vi "3_june.vi"() -> ()   [LabVIEW 2018]
uses:
  <vilib>/express/express analysis/Spectral/Block/exnSpectralBlock spectral measurements peak poly.vi
  <vilib>/express/express analysis/Spectral/Block/exnSpectralBlock spectral measurements peak DDT.vi
  <vilib>/express/express analysis/Spectral/XNode/ExpressSpectralMeasurementsBlockNode.xnode
panel:
  in  "stop (F)":bool
  out "Orignal Signal":dynamicdata(graph)
  in  "Threshold":dbl=0.1
  out "Portion":dynamicdata(graph)
  in  "Portion Duration":i32=200
  out "Index 0":dbl
  out "Index 1":dbl
  out "Index 2":dbl
  out "Index 3":dbl
  out "dt1":dbl
  out "dt2":dbl
  out "dt3":dbl
  in  "Manual depth":dbl=4.3
  in  "Mode":T1(ring)=enum."Use Far Field"
  out "x":dbl format="%#_6f"
  out "y":dbl format="%#_6f"
  out "z":dbl
  in  "peak min":dbl=0.1
  out "ratio":dbl
  out "ratio 2":dbl
  out "ratio 3":dbl
  out "ratio 4":dbl
  out "amplitude":dbl
  out "amplitude 2":dbl
  out "amplitude 3":dbl
  out "amplitude 4":dbl
  out "yaw":dbl
  out "pitch":dbl
  out "Yaw Chart":dbl(graph)
  out "Freq Domain":dynamicdata(graph)
  out "Ratio at Index (%)":dbl
  in  "LPF Cut-Off":dbl=40000.0 caption="Lower Cut-Off"
  out "Selected Index":i32
  in  "Operating Mode 2":T2(ring)=enum."Analyze Real-time"
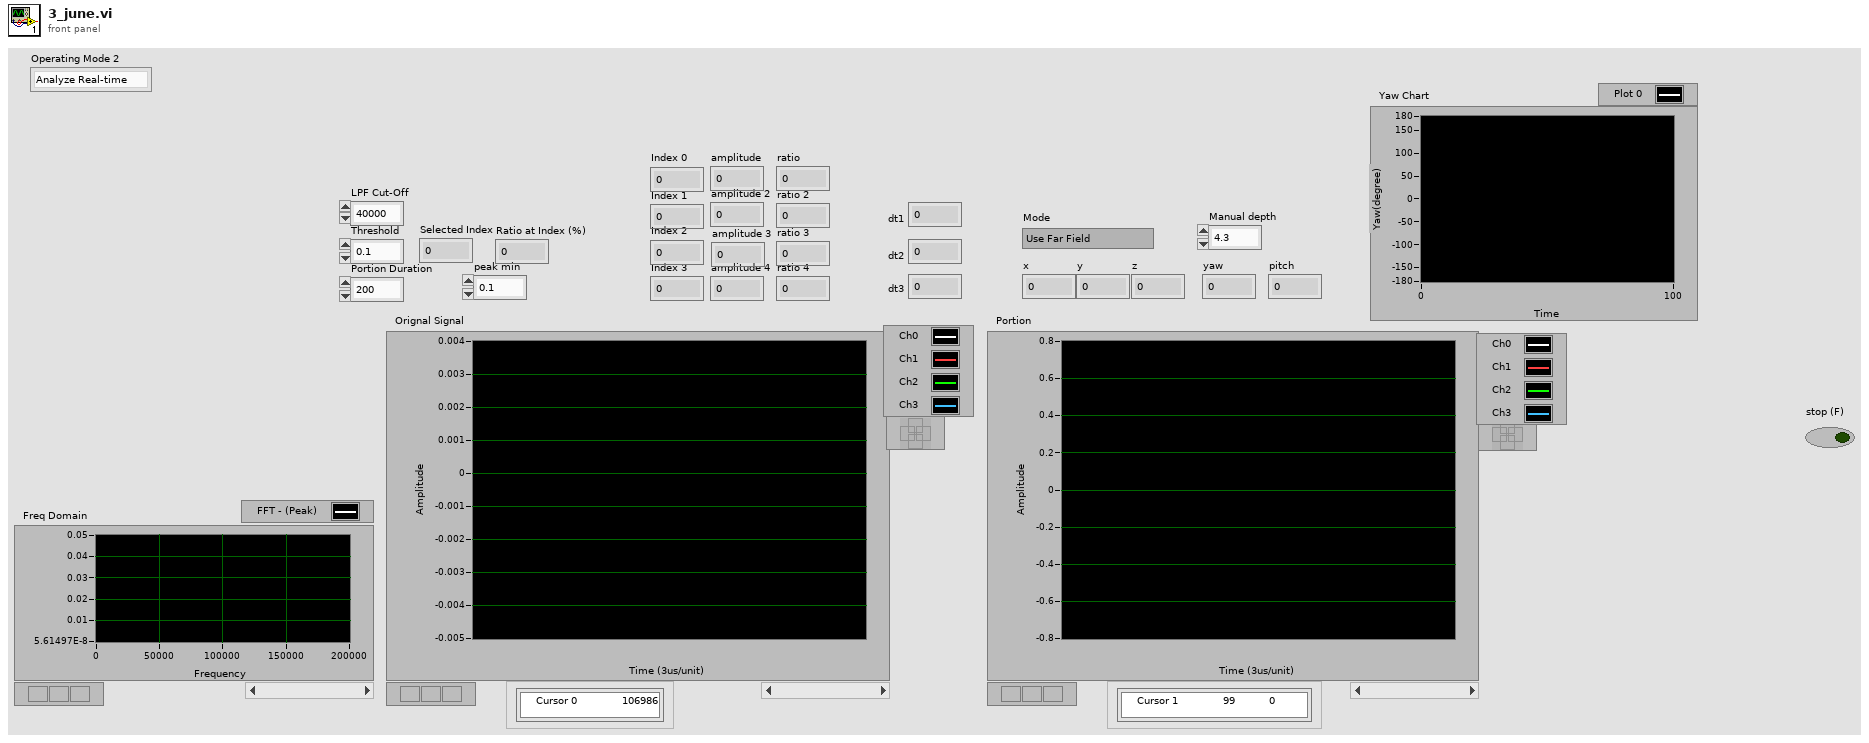
[diagram p1: front panel]
types:
  T1 = enum16{"Use Near Field", "Use Far Field", "Send to ROS", "Far Field with 3 hydrophones"}
  T2 = enum16{"Analyze From File", "Record Data", "Analyze Real-time"}
  T3 = cluster{"averaging mode":u16, "weighting mode":u16, "number of averages":u32}
  T4 = cluster{"dB On (F)":bool, "unwrap phase (F)":bool, "convert to degree (F)":bool}
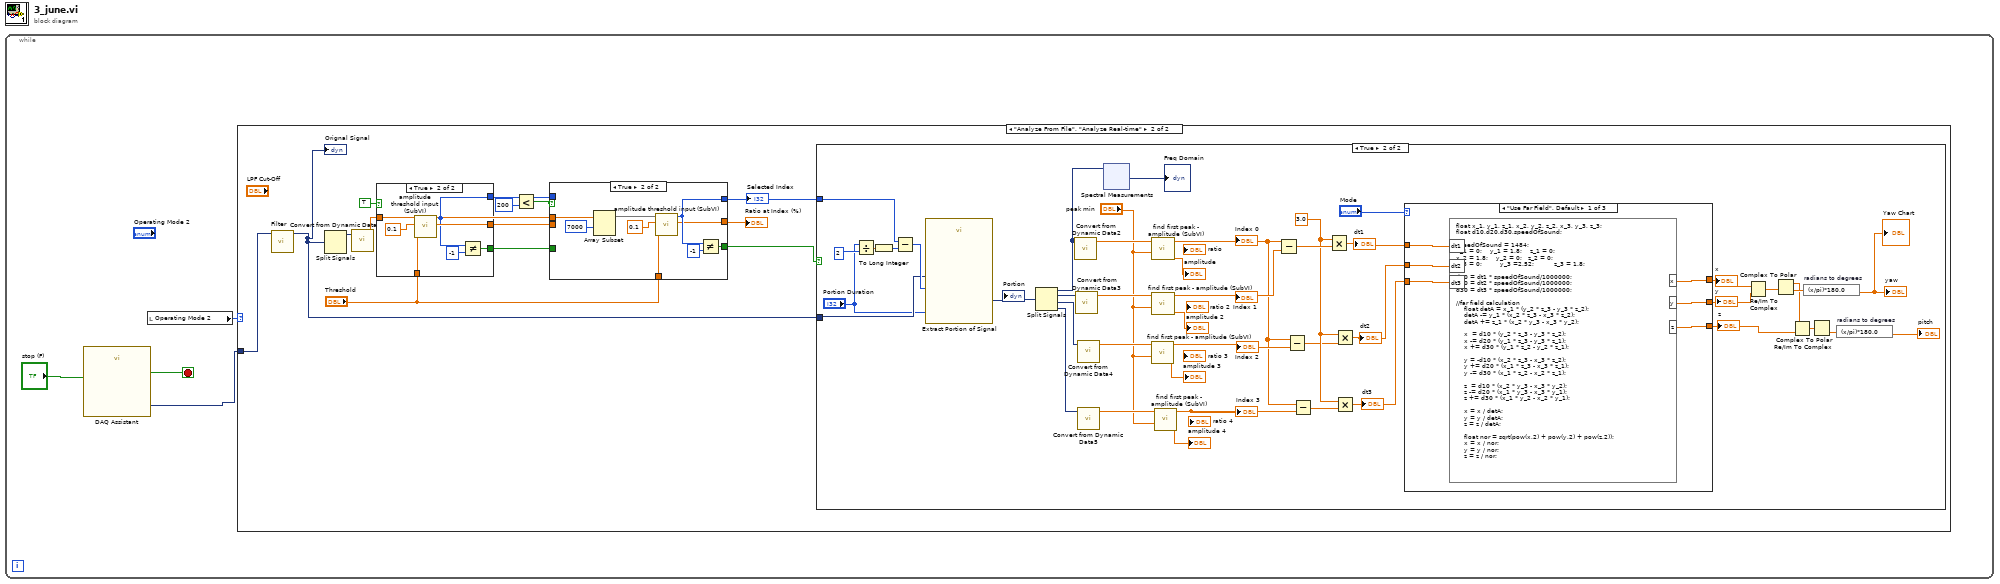
[diagram p0: block diagram]
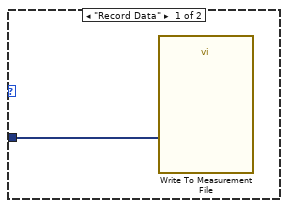
[diagram p2: hidden frame]
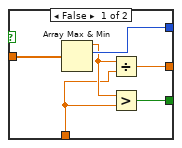
[diagram p4: hidden frame]
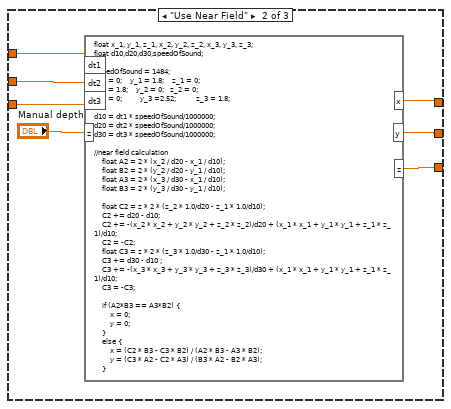
[diagram p6: hidden frame]
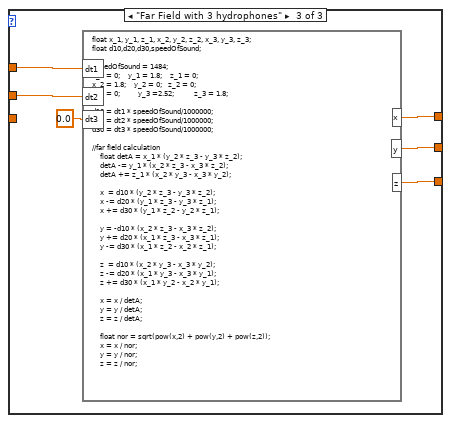
[diagram p7: hidden frame]
diagram:
  n1 = while {
    stop <- w4 stop-if-true
    n2 = call "DAQ Assistant"("stop (F)"="stop (F)") -> ("data"=w1:dynamicdata, "stopped"=w4:bool)  [unwired: 15 in, 2 out]
    n3 = local read "Operating Mode 2"() -> (w2:T2)
    n4 = case shown="\"Analyze From File\", \"Analyze Real-time\"" w2 {
      tunnel: w1 -> [w5 w8]
      frame "Record Data" {
        n5 = call "Write To Measurement File"("Signals"=w5) -> ()  [unwired: 16 in, 3 out]
      }
      frame "Analyze From File", "Analyze Real-time" {
        n6 = call "Filter"("Signal"=w8) -> ("Filtered Signal"=w6:dynamicdata)  [unwired: 9 in, 1 out]
        "Orignal Signal" <- w6
        n7 = Split Signals(w6) -> (w7:dynamicdata)  [unwired: 4 in, 3 out]
        n8 = call "Convert from Dynamic Data"("Dynamic Data Type"=w7) -> ("Array"=w14:dbl[])  [unwired: 3 in]
        n9 = case shown="True" TRUE {
          tunnel: w14 -> [w37 w44]
          tunnel: [w34 w41] -> w15
          tunnel: [w35 w40] -> w10
          tunnel: [w36 w39] -> w18
          tunnel: "Threshold" -> [w32 w38]
          frame False {
            n10 = Array Max & Min(array=w37) -> (max value=w33:dbl, max index (indices)=w35:i32)  [unwired: 2 out]
            n11 = Divide(x=w33, y=w32) -> (x/y=w34:dbl)
            n12 = Greater?(x=w33, y=w32) -> (0:w36:bool)
          }
          frame True {
            n13 = call "amplitude threshold input (SubVI).vi"("threshold"=w38, "%max amplitude"=0.1, "Array"=w44) -> ("actual ratio (%)"=w41:dbl, "Index"=w40:i32)  [unwired: 7 in]
            n14 = Not Equal?(x=w40, y=-1) -> (x != y?=w39:bool)
          }
        }
        n15 = Less?(x=w10, y=200) -> (x < y?=w16:bool)
        n16 = case shown="True" w16 {
          tunnel: w18 -> [w22 _]
          tunnel: w15 -> [w20 _]
          tunnel: w14 -> [_ w31]
          tunnel: "Threshold" -> [_ w26]
          tunnel: [w22 w25] -> w12
          tunnel: [w21 w24] -> w9
          tunnel: [w20 w23] -> w11
          tunnel: w10 -> [w21 _]
          frame False {
          }
          frame True {
            n17 = Array Subset(array=w31, index=7000) -> (w27:dbl[])  [unwired: 1 in]
            n18 = call "amplitude threshold input (SubVI).vi"("threshold"=w26, "%max amplitude"=0.1, "Array"=w27) -> ("actual ratio (%)"=w23:dbl, "Index"=w24:i32)  [unwired: 7 in]
            n19 = Not Equal?(x=w24, y=-1) -> (x != y?=w25:bool)
          }
        }
        "Ratio at Index (%)" <- w11
        "Selected Index" <- w9
        n20 = case shown="True" w12 {
          tunnel: w6 -> [_ w85]
          tunnel: w9 -> [_ w51]
          frame False {
          }
          frame True {
            w81 = 3.0 ("x")
            n21 = Divide(x="Portion Duration", y=2) -> (x/y=w55:dbl)
            n22 = To Long Integer(number=w55) -> (32bit integer=w54:i32)
            n23 = Subtract(x=w51, y=w54) -> (x-y=w88:i32)
            n24 = call "Extract Portion of Signal"("Samples"="Portion Duration", "Begin Sample"=w88, "Signals"=w85) -> ("Section"=w84:dynamicdata)  [unwired: 7 in, 1 out]
            "Portion" <- w84
            n25 = Split Signals(w84) -> (w45:dynamicdata, w87:dynamicdata, w86:dynamicdata, w83:dynamicdata)  [unwired: 4 in]
            n26 = call "Convert from Dynamic Data2"("Dynamic Data Type"=w45) -> ("Array"=w76:dbl[])  [unwired: 3 in]
            n27 = call "Convert from Dynamic Data3"("Dynamic Data Type"=w87) -> ("Array"=w75:dbl[])  [unwired: 3 in]
            n28 = call "Convert from Dynamic Data4"("Dynamic Data Type"=w86) -> ("Array"=w74:dbl[])  [unwired: 3 in]
            n29 = call "Convert from Dynamic Data5"("Dynamic Data Type"=w83) -> ("Array"=w73:dbl[])  [unwired: 3 in]
            n30 = xnode "Spectral Measurements"("Signals"=w45) -> ("FFT - (Peak)"=→"Freq Domain":dynamicdata)  [unwired: 1 in, 2 out]
            n31 = call "find first peak - amplitude (SubVI).vi"("threshold ratio"="peak min", "Array"=w74) -> ("Peak threshold"=→"amplitude 3":dbl, "Index"=w71:dbl)  [unwired: 5 in, 3 out]
            "Index 2" <- w71
            n32 = call "find first peak - amplitude (SubVI).vi"("threshold ratio"="peak min", "Array"=w76) -> ("Peak threshold"=→"amplitude":dbl, "Index"=w70:dbl)  [unwired: 5 in, 3 out]
            "Index 0" <- w70
            n33 = call "find first peak - amplitude (SubVI).vi"("threshold ratio"="peak min", "Array"=w75) -> ("Peak threshold"=→"amplitude 2":dbl, "Index"=w72:dbl)  [unwired: 5 in, 3 out]
            "Index 1" <- w72
            n34 = call "find first peak - amplitude (SubVI).vi"("threshold ratio"="peak min", "Array"=w73) -> ("Peak threshold"=→"amplitude 4":dbl, "Index"=w69:dbl)  [unwired: 5 in, 3 out]
            "Index 3" <- w69
            n35 = Subtract(x=w70, y=w72) -> (x-y=w82:dbl)
            n36 = Subtract(x=w70, y=w71) -> (x-y=w80:dbl)
            n37 = Subtract(x=w70, y=w69) -> (x-y=w79:dbl)
            n38 = Multiply(x=w81, y=w82) -> (x*y=w58:dbl)
            "dt1" <- w58
            n39 = Multiply(x=w81, y=w80) -> (x*y=w78:dbl)
            "dt2" <- w78
            n40 = Multiply(x=w81, y=w79) -> (x*y=w57:dbl)
            "dt3" <- w57
            n41 = case shown="\"Use Far Field\", Default" "Mode" {
              tunnel: w58 -> [w104 w111 w117]
              tunnel: w78 -> [w103 w110 w116]
              tunnel: [w102 w109 w114] -> w65
              tunnel: [w101 w108 w113] -> w64
              tunnel: [w100 w107 w112] -> w63
              tunnel: w57 -> [w99 w105 _]
              frame "Use Far Field", Default {
                n42 = formula code="float x_1, y_1, z_1, x_2, y_2, z_2, x_3, y_3, z_3;\nfloat d10,d20,d30,speedOfSound;\n\nspeedOfSound = 1484;\nx_1 = 0;    y_1 = 1.8;    z_1 = 0;\nx_2 = 1.8;    y_2 = 0;   z_2 = 0;\nx_3 = 0;         y_3 =2.52;          z_3 = 1.8;\n\nd10 = dt1 * speedOfSound/1000000;\nd20 = dt2 * speedOfSound/1000000;\nd30 = dt3 * speedOfSound/1000000;\n\n//far field calculation\n    float detA = x_1 * (y_2 * z_3 - y_3 * z_2);\n    detA -= y_1 * (x_2 * z_3 - x_3 * z_2);\n    detA += z_1 * (x_2 * y_3 - x_3 * y_2);\n\n    x  = d10 * (y_2 * z_3 - y_3 * z_2);\n    x -= d20 * (y_1 * z_3 - y_3 * z_1);\n    x += d30 * (y_1 * z_2 - y_2 * z_1);\n\n    y = -d10 * (x_2 * z_3 - x_3 * z_2);\n    y += d20 * (x_1 * z_3 - x_3 * z_1);\n    y -= d30 * (x_1 * z_2 - x_2 * z_1);\n\n    z  = d10 * (x_2 * y_3 - x_3 * y_2);\n    z -= d20 * (x_1 * y_3 - x_3 * y_1);\n    z += d30 * (x_1 * y_2 - x_2 * y_1);\n\n    x = x / detA;\n    y = y / detA;\n    z = z / detA;\n\n    float nor = sqrt(pow(x,2) + pow(y,2) + pow(z,2));\n    x = x / nor;\n    y = y / nor;\n    z = z / nor;"("dt1"=w104, "dt2"=w103, "dt3"=w99) -> ("x"=w102:dbl, "y"=w101:dbl, "z"=w100:dbl)
              }
              frame "Use Near Field" {
                n43 = formula code="float x_1, y_1, z_1, x_2, y_2, z_2, x_3, y_3, z_3;\nfloat d10,d20,d30,speedOfSound;\n\nspeedOfSound = 1484;\nx_1 = 0;    y_1 = 1.8;    z_1 = 0;\nx_2 = 1.8;    y_2 = 0;   z_2 = 0;\nx_3 = 0;         y_3 =2.52;          z_3 = 1.8;\n\nd10 = dt1 * speedOfSound/1000000;\nd20 = dt2 * speedOfSound/1000000;\nd30 = dt3 * speedOfSound/1000000;\n\n//near field calculation\n    float A2 = 2 * (x_2 / d20 - x_1 / d10);\n    float B2 = 2 * (y_2 / d20 - y_1 / d10);\n    float A3 = 2 * (x_3 / d30 - x_1 / d10);\n    float B3 = 2 * (y_3 / d30 - y_1 / d10);\n    \n    float C2 = z * 2 * (z_2 * 1.0/d20 - z_1 * 1.0/d10);\n    C2 += d20 - d10;\n    C2 += -(x_2 * x_2 + y_2 * y_2 + z_2 * z_2)/d20 + (x_1 * x_1 + y_1 * y_1 + z_1 * z_1)/d10;\n    C2 = -C2;\n    float C3 = z * 2 * (z_3 * 1.0/d30 - z_1 * 1.0/d10);\n    C3 += d30 - d10 ;\n    C3 += -(x_3 * x_3 + y_3 * y_3 + z_3 * z_3)/d30 + (x_1 * x_1 + y_1 * y_1 + z_1 * z_1)/d10;\n    C3 = -C3;\n\n    if (A2*B3 == A3*B2) {\n        x = 0;\n        y = 0;\n    }\n    else {\n        x = (C2 * B3 - C3 * B2) / (A2 * B3 - A3 * B2);\n        y = (C3 * A2 - C2 * A3) / (B3 * A2 - B2 * A3);\n    }"("dt1"=w111, "dt2"=w110, "dt3"=w105, "z"="Manual depth") -> ("x"=w109:dbl, "y"=w108:dbl, "z"=w107:dbl)
              }
              frame "Far Field with 3 hydrophones" {
                n44 = formula code="float x_1, y_1, z_1, x_2, y_2, z_2, x_3, y_3, z_3;\nfloat d10,d20,d30,speedOfSound;\n\nspeedOfSound = 1484;\nx_1 = 0;    y_1 = 1.8;    z_1 = 0;\nx_2 = 1.8;    y_2 = 0;   z_2 = 0;\nx_3 = 0;         y_3 =2.52;          z_3 = 1.8;\n\nd10 = dt1 * speedOfSound/1000000;\nd20 = dt2 * speedOfSound/1000000;\nd30 = dt3 * speedOfSound/1000000;\n\n//far field calculation\n    float detA = x_1 * (y_2 * z_3 - y_3 * z_2);\n    detA -= y_1 * (x_2 * z_3 - x_3 * z_2);\n    detA += z_1 * (x_2 * y_3 - x_3 * y_2);\n\n    x  = d10 * (y_2 * z_3 - y_3 * z_2);\n    x -= d20 * (y_1 * z_3 - y_3 * z_1);\n    x += d30 * (y_1 * z_2 - y_2 * z_1);\n\n    y = -d10 * (x_2 * z_3 - x_3 * z_2);\n    y += d20 * (x_1 * z_3 - x_3 * z_1);\n    y -= d30 * (x_1 * z_2 - x_2 * z_1);\n\n    z  = d10 * (x_2 * y_3 - x_3 * y_2);\n    z -= d20 * (x_1 * y_3 - x_3 * y_1);\n    z += d30 * (x_1 * y_2 - x_2 * y_1);\n\n    x = x / detA;\n    y = y / detA;\n    z = z / detA;\n\n    float nor = sqrt(pow(x,2) + pow(y,2) + pow(z,2));\n    x = x / nor;\n    y = y / nor;\n    z = z / nor;"("dt1"=w117, "dt2"=w116, "dt3"=0.0 ("input variable")) -> ("x"=w114:dbl, "y"=w113:dbl, "z"=w112:dbl)
              }
            }
            "x" <- w65
            "y" <- w64
            "z" <- w63
            n45 = Re/Im To Complex(1:w64, 2:w65) -> (0:w67:cdb)
            n46 = Complex To Polar(r * e^(i*theta)=w67) -> (r=w62:dbl, theta=w66:dbl)
            n47 = Re/Im To Complex(1:w63, 2:w62) -> (0:w61:cdb)
            n48 = expression code="(x/pi)*180.0" "radians to degrees"(w66) -> (→"yaw" →"Yaw Chart":dbl)
            n49 = Complex To Polar(r * e^(i*theta)=w61) -> (theta=w59:dbl)  [unwired: 1 out]
            n50 = expression code="(x/pi)*180.0" "radians to degrees"(w59) -> (→"pitch":dbl)
          }
        }
      }
    }
  }
